vi "ModifyClassAttribute.vi"(1 "Lock time (ms)":u32, 5 "error in (no error)":errorcluster) -> (16 "created new":bool, 19 "error out":errorcluster)   [LabVIEW 2017, in "G#BaseClass1.lvclass"]
uses:
  G#BaseClass1.lvclass
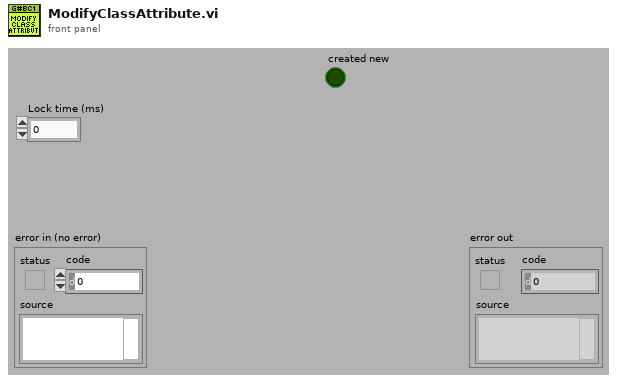
[diagram p1: front panel]
types:
  T1 = typedef "G#BaseClass1.lvclass/ClassAttributesRef.ctl" = refnum<data-value>
  T2 = typedef "G#BaseClass1.lvclass/ClassAttributes.ctl" = cluster{"Int":i32, "ArrayInt":i32[]}
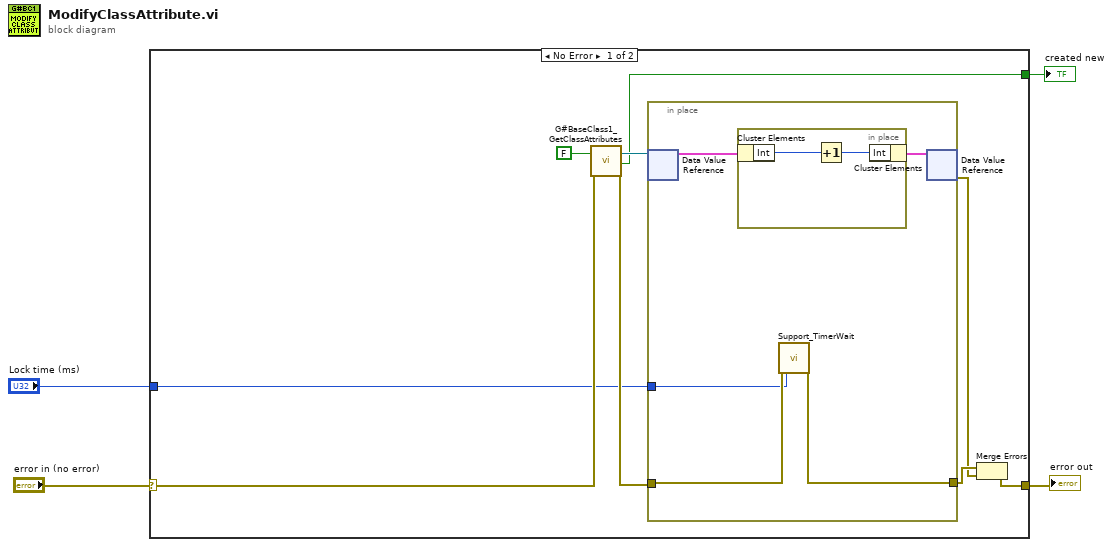
[diagram p0: block diagram]
diagram:
  n1 = case shown="No Error" "error in (no error)" {
    selector: "error in (no error)" -> [w13 w21]
    tunnel: [w10 w21] -> w3
    tunnel: "Lock time (ms)" -> [w6 _]
    tunnel: [w5 _] -> w1
    frame No Error {
      n2 = call "G#BaseClass1_GetClassAttributes.vi"("return data? (T)"=FALSE ("return data"), "error in (no error)"=w13) -> ("class attributes ref"=w11:T1, "created new?"=w5:bool, "error out"=w12:errorcluster)  [unwired: 14 in, 1 out]
      n3 = in-place {
        in-place-border: w12 -> [w16]
        in-place-border: [w15] -> w8
        in-place-border: w6 -> [w14]
        n4 = in-place-dvr #1(w11) -> (w17:T2)  [unwired: 1 out]
        n5 = in-place {
          n6 = in-place-cluster #2(w17) -> ("Int"=w20:i32)
          n7 = Increment(x=w20) -> (x+1=w19:i32)
          n8 = in-place-cluster #2("Int"=w19) -> (w18:T2)
        }
        n9 = call "Support_TimerWait.vi"("error in (no error)"=w16, "milliseconds to wait"=w14) -> ("error out"=w15:errorcluster)  [unwired: 17 in]
        n10 = in-place-dvr #1(w18) -> (w7:errorcluster)  [unwired: 1 out]
      }
      n11 = Merge Errors(w8, w7) -> (w10:errorcluster)
    }
    frame Error {
    }
  }
  "error out" <- w3
  "created new" <- w1
